vi "Rectify.vi"(7 "Max Value":dbl=1.0, 11 "Value":dbl) -> (3 "Rectified":dbl)   [LabVIEW 2013]
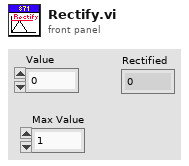
[diagram p1: front panel]
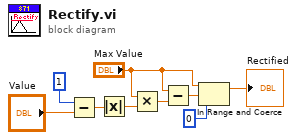
[diagram p0: block diagram]
diagram:
  n1 = Subtract(x=1, y="Value") -> (x-y=w8:dbl)
  n2 = Absolute Value(x=w8) -> (abs(x)=w7:dbl)
  n3 = Multiply(x="Max Value", y=w7) -> (x*y=w6:dbl)
  n4 = Subtract(x="Max Value", y=w6) -> (x-y=w5:dbl)
  n5 = In Range and Coerce(upper limit="Max Value", x=w5, lower limit=0) -> (coerced(x)=→"Rectified":dbl)  [unwired: 1 out]
